vi "EstimateAcqTime.vi"(9 "ExpIncreaseEn?":bool=TRUE, 11 "Config":T1 {"Hardware Configuration"."Lasers Configuration"."SettingValues"."785 Power" format="%.1f"; "Hardware Configuration"."Lasers Configuration"."SettingValues"."647 Power" format="%.1f"; "Hardware Configuration"."Lasers Configuration"."SettingValues"."561 Power" format="%.1f"}) -> (1 "AcqTime/ms":dbl, 2 "AcqTime/min":dbl, 3 "Config 2":T1 {"Hardware Configuration"."Lasers Configuration"."SettingValues"."785 Power" format="%.1f"; "Hardware Configuration"."Lasers Configuration"."SettingValues"."647 Power" format="%.1f"; "Hardware Configuration"."Lasers Configuration"."SettingValues"."561 Power" format="%.1f"})   [LabVIEW 2020]
uses:
  Settings/System Running Settings.ctl
  Support/Hardware Configuration.ctl
  Support/Camera Configuration.ctl
  controls/ROI.ctl
  D:/Daguan/Development/RM21-MMicrosopeSource/HardwareAdapter/Camera/Dependencies/PVCamNET.dll
  Dependencies/PVCamNET.dll
  <vilib>/vision/Image Controls.llb/IMAQ Image.ctl
  D:/Daguan/Development/RM21-MMicrosopeSource/HardwareAdapter/Lasers/Dependencies/Oxxius_Boxx.dll
  Lasers/Dependencies/Oxxius_Boxx.dll
  Logging/Logging Configuration.ctl
  controls/DeviceStatusCtl.ctl
  controls/CallBack Refs.ctl
  Logging/Logging.lvlib
  Settings/Settings.lvlib
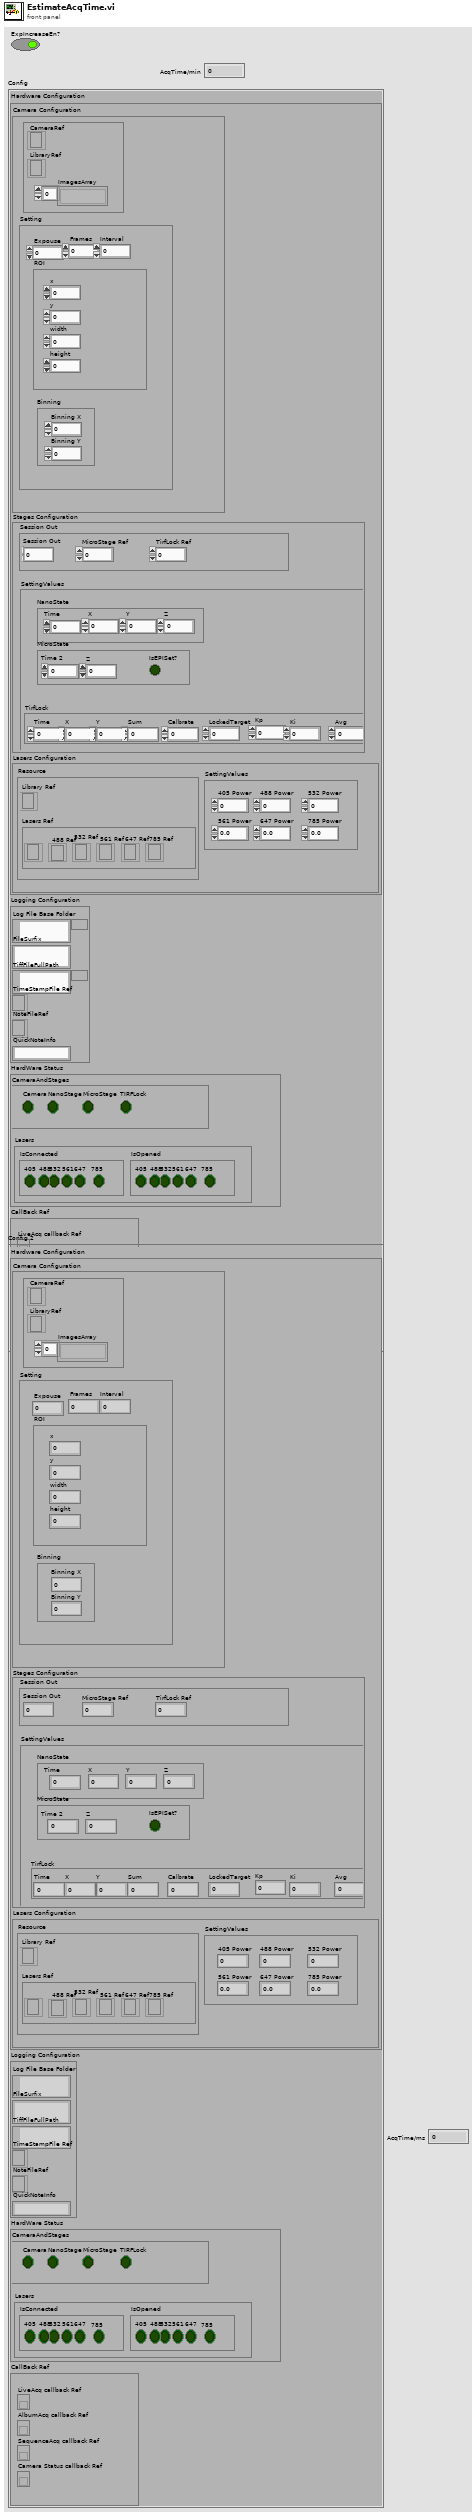
[diagram p1: front panel]
types:
  T1 = typedef "Settings.lvlib/System Running Settings.ctl" = cluster{"Hardware Configuration":T2, "Logging Configuration":T6, "HardWare Status":cluster{"CameraAndStages":T7, "Lasers":cluster{"IsConnected":cluster{"405":bool, "488":bool, "532":bool, "561":bool, "647":bool, "785":bool}, "IsOpened":cluster{"405":bool, "488":bool, "532":bool, "561":bool, "647":bool, "785":bool}}}, "CallBack Ref":T8}
  T2 = typedef "Hardware Configuration.ctl" = cluster{"Camera Configuration":T3, "Stages Configuration":cluster{"Resource":cluster{"NanoStage Ref":i32, "MicroStage Ref":i32, "TirfLock Ref":i32}, "SettingValues":cluster{"NanoState":cluster{"Time":dbl, "X":dbl, "Y":dbl, "Z":dbl}, "MicroState":cluster{"Time 2":dbl, "Z":dbl, "IsEPISet?":bool}, "TirfLock":cluster{"Time":dbl, "X":dbl, "Y":dbl, "Sum":dbl, "Calbrate":dbl, "LockedTarget":dbl, "Kp":dbl, "Ki":dbl, "Avg":dbl}}}, "Lasers Configuration":cluster{"SettingValues":cluster{"405 Power":sgl, "488 Power":sgl, "532 Power":sgl, "561 Power":sgl, "647 Power":sgl, "785 Power":sgl}, "Resource":cluster{"Library Ref":refnum<k24>, "Lasers Ref":cluster{"405 Ref":refnum<k24>, "488 Ref":refnum<k24>, "532 Ref":refnum<k24>, "561 Ref":refnum<k24>, "647 Ref":refnum<k24>, "785 Ref":refnum<k24>}}}}
  T3 = typedef "Camera Configuration.ctl" = cluster{"Setting":cluster{"Expouse":dbl, "Frames":dbl, "Interval":dbl, "ROI":T4, "Binning":cluster{"Binning X":dbl, "Binning Y":dbl}}, "Resource":cluster{"CameraRef":refnum<k24>, "LibraryRef":refnum<k24>, "ImagesArray":T5[]}}
  T4 = typedef "ROI.ctl" = cluster{"x":dbl, "y":dbl, "width":dbl, "height":dbl}
  T5 = typedef "IMAQ Image.ctl" = refnum<image>
  T6 = typedef "Logging.lvlib/Logging Configuration.ctl" = cluster{"Log File Base Folder":path, "FileSurfix":string, "TiffFileFullPath":path, "TimeStampFile Ref":refnum<file>, "NoteFileRef":refnum<file>, "QuickNoteInfo":string}
  T7 = typedef "DeviceStatusCtl.ctl" = cluster{"Camera":bool, "NanoStage":bool, "MicroStage":bool, "TIRFLock":bool}
  T8 = typedef "CallBack Refs.ctl" = cluster{"LiveAcq callback Ref":refnum<k27>, "AlbumAcq callback Ref":refnum<k27>, "SequenceAcq callback Ref":refnum<k27>, "Camera Status callback Ref":refnum<k27>}
  T9 = cluster{"Expouse":dbl, "Frames":dbl, "Interval":dbl, "ROI":T4, "Binning":cluster{"Binning X":dbl, "Binning Y":dbl}}
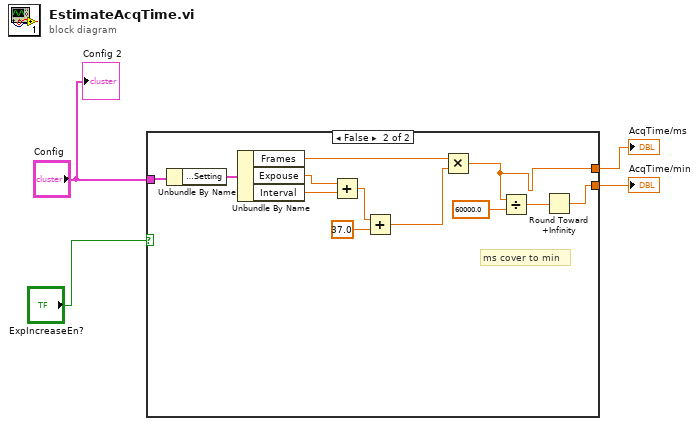
[diagram p0: block diagram]
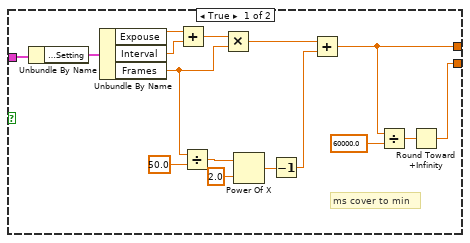
[diagram p2: hidden frame]
diagram:
  n1 = case shown="False" "ExpIncreaseEn?" {
    tunnel: "Config" -> [w20 w32]
    tunnel: [w12 w25] -> w4
    tunnel: [w11 w24] -> w1
    frame True {
      # "ms cover to min"
      n2 = Unbundle By Name(w20) -> ("Hardware Configuration.Camera Configuration.Setting"=w19:T9)
      n3 = Unbundle By Name(w19) -> ("Expouse"=w9:dbl, "Interval"=w8:dbl, "Frames"=w6:dbl)
      n4 = Add(x=w9, y=w8) -> (x+y=w7:dbl)
      n5 = Divide(x=w6, y=50.0) -> (x/y=w16:dbl)
      n6 = Multiply(x=w7, y=w6) -> (x*y=w5:dbl)
      n7 = Power Of X(1:2.0 ("x"), 2:w16) -> (0:w17:dbl)
      n8 = Decrement(x=w17) -> (x-1=w10:dbl)
      n9 = Add(x=w5, y=w10) -> (x+y=w11:dbl)
      n10 = Divide(x=w11, y=60000.0) -> (x/y=w13:dbl)
      n11 = Round Toward +Infinity(x=w13) -> (ceil(x): smallest int >= x=w12:dbl)
    }
    frame False {
      # "ms cover to min"
      n12 = Unbundle By Name(w32) -> ("Hardware Configuration.Camera Configuration.Setting"=w31:T9)
      n13 = Unbundle By Name(w31) -> ("Frames"=w28:dbl, "Expouse"=w30:dbl, "Interval"=w29:dbl)
      n14 = Add(x=w30, y=w29) -> (x+y=w23:dbl)
      n15 = Add(x=w23, y=37.0) -> (x+y=w22:dbl)
      n16 = Multiply(x=w28, y=w22) -> (x*y=w24:dbl)
      n17 = Divide(x=w24, y=60000.0) -> (x/y=w26:dbl)
      n18 = Round Toward +Infinity(x=w26) -> (ceil(x): smallest int >= x=w25:dbl)
    }
  }
  "AcqTime/min" <- w4
  "AcqTime/ms" <- w1
  "Config 2" <- "Config"
